vi "Remove_Spikes_sub.vi"(8 "Number of Sigma to cut after":dbl=3.0, 9 "Number of samples":i32, 10 "Time Trace in":dbl[](array[numeric]), 11 "Bkgnd Variance":dbl) -> (0 "Checked":bool, 2 "Time Trace out":dbl[](array[numeric]), 3 "Numeric out":i32)   [LabVIEW 2014]
uses:
  <vilib>/Analysis/NI_AALBase.lvlib
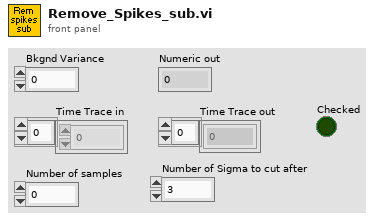
[diagram p1: front panel]
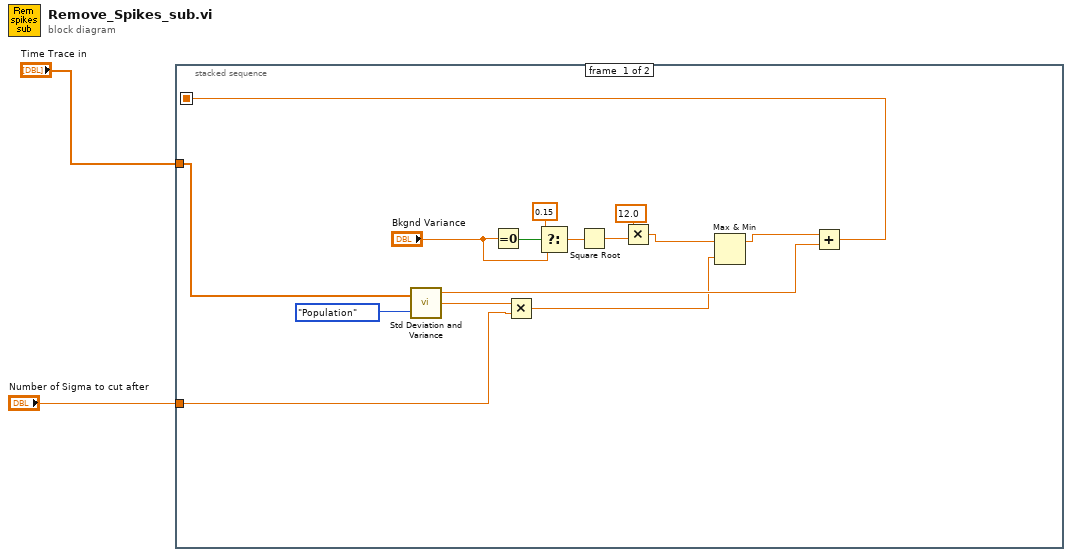
[diagram p0: block diagram]
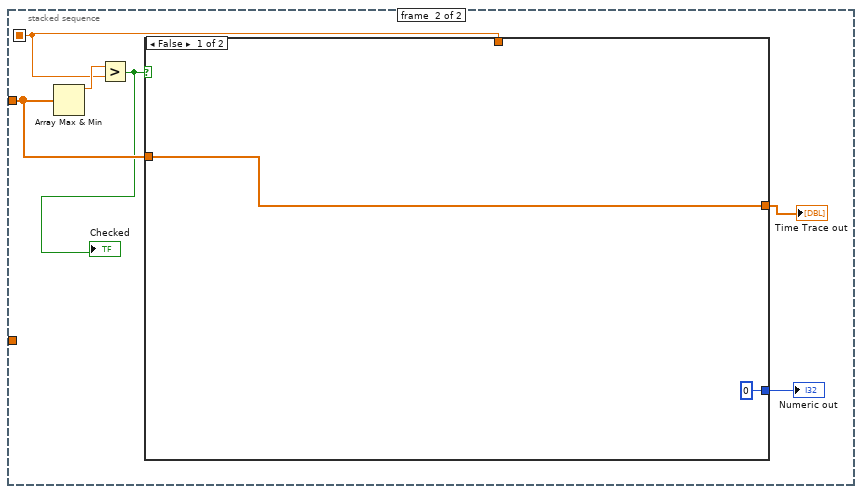
[diagram p2: hidden frame]
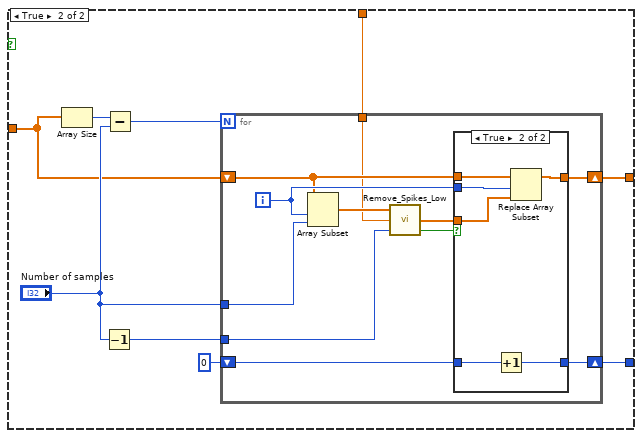
[diagram p3: hidden frame]
diagram:
  n1 = stacked-sequence {
    seq-local: [w9 _] -> [_ w19]
    tunnel: "Time Trace in" -> [w10 w20]
    tunnel: "Number of Sigma to cut after" -> [w3 _]
    frame #0 {
      n2 = call <vilib>:"Std Deviation and Variance.vi"("X"=w10, "Weighting (Sample)"=enum16{"Sample", "Population"}."Population") -> ("mean"=w13:dbl, "standard deviation"=w7:dbl)  [unwired: 1 out]
      n3 = Equal To 0?(x="Bkgnd Variance") -> (x = 0?=w17:bool)
      n4 = Multiply(x=w7, y=w3) -> (x*y=w5:dbl)
      n5 = Select(t=0.15, s=w17, f="Bkgnd Variance") -> (s? t:f=w15:dbl)
      n6 = Square Root(x=w15) -> (sqrt(x)=w12:dbl)
      n7 = Multiply(x=12.0 ("y"), y=w12) -> (x*y=w6:dbl)
      n8 = Max & Min(x=w6, y=w5) -> (max(x,y)=w4:dbl)  [unwired: 1 out]
      n9 = Add(x=w4, y=w13) -> (x+y=w9:dbl)
    }
    frame #1 {
      n10 = Array Max & Min(array=w20) -> (max value=w21:dbl)  [unwired: 3 out]
      n11 = Greater?(x=w21, y=w19) -> (0:w18:bool)
      "Checked" <- w18
      n12 = case shown="False" w18 {
        tunnel: [0 w32] -> w23
        tunnel: [w25 w31] -> w22
        tunnel: w19 -> [_ w27]
        tunnel: w20 -> [w25 w26]
        frame False {
        }
        frame True {
          n13 = Array Size(array=w26) -> (size(s)=w29:i32)
          n14 = Decrement(x="Number of samples") -> (x-1=w28:i32)
          n15 = Subtract(x=w29, y="Number of samples") -> (x-y=w30:i32)
          n16 = for {
            N: w30 -> [_]
            shift-right: [w38] -> w31
            shift-left: w26 -> [w39]
            tunnel: "Number of samples" -> [w45]
            tunnel: w28 -> [w44]
            tunnel: w27 -> [w37]
            shift-right: [w36] -> w32
            shift-left: 0 -> [w35]
            i -> [w41]
            n17 = Array Subset(array=w39, index=w41, length=w45) -> (w43:dbl[])
            n18 = call "Remove_Spikes_Low.vi"("index"=w44, "Background noise"=w37, "Time Trace"=w43) -> ("Spike"=w42:bool, "Filtered Time Trace"=w40:dbl[])  [unwired: 1 out]
            n19 = case shown="True" w42 {
              tunnel: w41 -> [_ w53]
              tunnel: w40 -> [_ w52]
              tunnel: w39 -> [w47 w51]
              tunnel: [w47 w50] -> w38
              tunnel: [w46 w48] -> w36
              tunnel: w35 -> [w46 w49]
              frame False {
              }
              frame True {
                n20 = Increment(x=w49) -> (x+1=w48:i32)
                n21 = Replace Array Subset(array=w51, new element=w52, index=w53) -> (w50:dbl[])
              }
            }
          }
        }
      }
      "Numeric out" <- w23
      "Time Trace out" <- w22
    }
  }
